vi "timing_channel_path.get.vi"(8 "error in (no error)":errorcluster, 11 "Item Ref in":T1 format="%.0x") -> (0 "error out":errorcluster, 2 "Timing Channel Path":string, 3 "Item Ref out":T1=18446744073709551615 format="%.0x")   [LabVIEW 2024, in "Nominal Client Scripting.lvlib"]
uses:
  <vilib>/NI VeriStand/Custom Device API/Custom Device Item Ref.ctl
  Nominal Client Scripting.lvlib
  <vilib>/NI VeriStand/Custom Device API/Custom Device API.lvlib
  <vilib>/NI VeriStand/Custom Device API/Get Item Property (String).vi
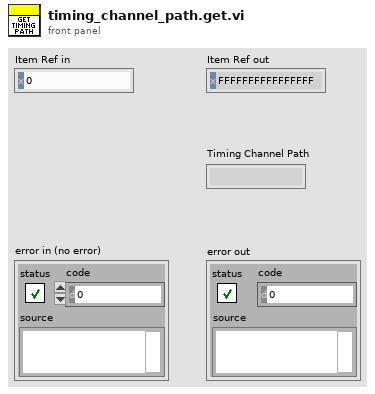
[diagram p1: front panel]
types:
  T1 = typedef "Custom Device API.lvlib/Custom Device Item Ref.ctl" = u64
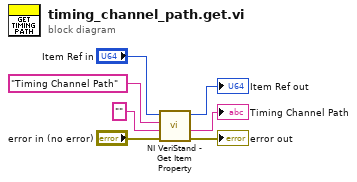
[diagram p0: block diagram]
diagram:
  n1 = call-poly <vilib>:"NI VeriStand - Get Item Property.vi"("error in (no error)"="error in (no error)", "Default Value"="", "Property Name"="Timing Channel Path", "Item Ref in"="Item Ref in") -> ("error out"=→"error out":errorcluster, "Value"=→"Timing Channel Path":string, "Item Ref out"=→"Item Ref out":T1)  [unwired: 4 in, 1 out]
